vi "Test Set-Point Driver Function.vi"() -> (0 "Reason":string, 1 "Success":bool)   [LabVIEW 2013]
uses:
  <vilib>/xml/Load XML File.vi
  <vilib>/xml/NI_XML.lvlib
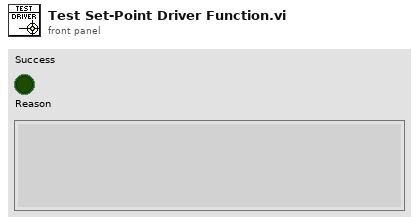
[diagram p1: front panel]
types:
  T1 = typedef "Sidecar Debug Queue.ctl" = refnum<queue>
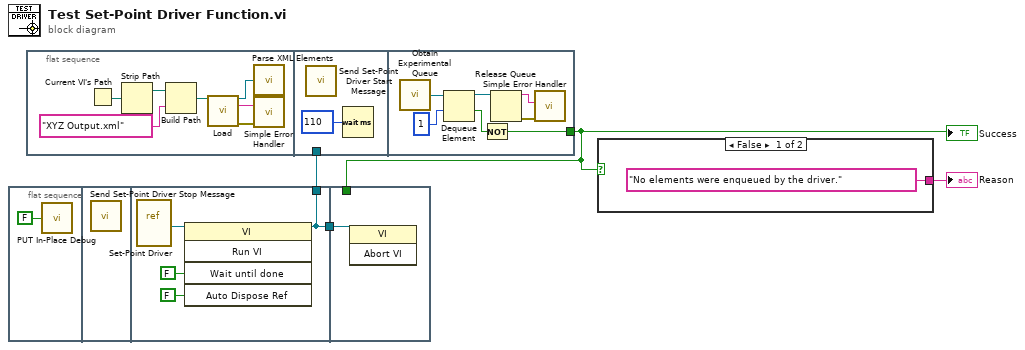
[diagram p0: block diagram]
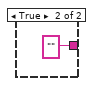
[diagram p2: hidden frame]
diagram:
  n1 = flat-sequence {
    tunnel: [w6] -> w3
    tunnel: [w6] -> w2
    tunnel: w3 -> [w10]
    tunnel: w1 -> [_]
    frame #0 {
      n2 = call "PUT In-Place Debug.vi"("In Place Debug Enabled"=FALSE) -> ()
    }
    frame #1 {
      n3 = call "Send Set-Point Driver Stop Message.vi"() -> ()  [unwired: 1 in]
    }
    frame #2 {
      n4 = vi-ref "Set-Point Driver.vi"() -> (w9:refnum<vi>)
      n5 = invoke class="VI" method="Run VI"(reference=w9, "Wait until done"=FALSE ("Wait Until Done"), "Auto Dispose Ref"=FALSE ("Auto Dispose Reference")) -> (reference out=w6:refnum<vi>)  [unwired: 2 in, 4 out]
    }
    frame #3 {
      n6 = invoke class="VI" method="Abort VI"(reference=w10) -> ()  [unwired: 2 in, 3 out]
    }
  }
  n7 = flat-sequence {
    tunnel: w2 -> [_]
    tunnel: [w19] -> w1
    frame #0 {
      n8 = Current VI's Path() -> (path=w17:path)
      n9 = Strip Path(path=w17) -> (stripped path=w16:path)  [unwired: 1 out]
      n10 = Build Path(base path=w16, name or relative path="XYZ Output.xml") -> (appended path=w11:path)
      n11 = call-poly <vilib>:"Load.vi"("path to XML document"=w11) -> ("DOM document out"=w14:refnum<k20>, "parse errors"=w12:string, "error out"=w13:errorcluster)  [unwired: 12 in]
      n12 = call "Parse XML Elements.vi"("DOM"=w14) -> ()
      n13 = call <vilib>:"Simple Error Handler.vi"("error source (\" \")"=w12, "error in (no error)"=w13) -> ()  [unwired: 3 in, 5 out]
    }
    frame #1 {
      n14 = call "Send Set-Point Driver Start Message.vi"() -> ()  [unwired: 1 in]
      n15 = Wait (ms)(milliseconds to wait=u32 110) -> ()  [unwired: 1 out]
    }
    frame #2 {
      n16 = call "Obtain Experimental Queue.vi"() -> ("Queue"=w24:T1)
      n17 = Dequeue Element(queue=w24, timeout in ms (-1)=1) -> (queue out=w23:T1, timed out?=w20:bool)  [unwired: 1 in, 2 out]
      n18 = Not(x=w20) -> (.not. x?=w19:bool)
      n19 = Release Queue(queue=w23) -> (queue name=w22:string, error out=w21:errorcluster)  [unwired: 2 in, 1 out]
      n20 = call <vilib>:"Simple Error Handler.vi"("error source (\" \")"=w22, "error in (no error)"=w21) -> ()  [unwired: 3 in, 5 out]
    }
  }
  n21 = case shown="False" w1 {
    tunnel: ["No elements were enqueued by the driver." ("name or relative path") "" ("name or relative path")] -> w4
    frame False {
    }
    frame True {
    }
  }
  "Reason" <- w4
  "Success" <- w1
